vi "Msg To.vi"(9 "Event Actor":refnum<class "Event Actor.lvclass">, 10 "Alias":string) -> (3 "Event Create Msg out":refnum<class "Event Create Msg.lvclass">)   [LabVIEW 2021, in "Event Create.lvlib" / "Event Create Msg.lvclass"]
uses:
  Event Create Msg.lvclass
  Event Create Msg.lvclass/Event Create Msg.ctl
  Event Actor/Event Actor.lvclass
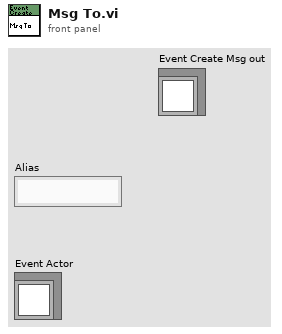
[diagram p1: front panel]
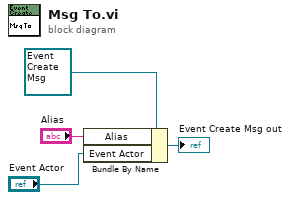
[diagram p0: block diagram]
diagram:
  n1 = Bundle By Name(cluster=refnum<class "Event Create Msg.lvclass"> refnum ("Event Create Msg out"), "Alias"="Alias", "Event Actor"="Event Actor") -> (→"Event Create Msg out":refnum<class "Event Create Msg.lvclass">)
